vi "Report read csv G.vi"(2 "error in":errorcluster) -> (0 "error out":errorcluster)   [LabVIEW 2015]
uses:
  <vilib>/Utility/file.llb/Read Delimited Spreadsheet (string).vi
  <vilib>/Utility/miscctls.llb/LVRowAndColumnTypeDef.ctl
panel:
  out "Table Control":string[][](table)
  in  "Exit":bool
  in  "Select Date":u16(ring) items=["Select Date", "10_07_20.csv"]
  in  "Select Model No":u16(ring) items=["Select Model", "Global", "Medium"]
  # "Report Data"
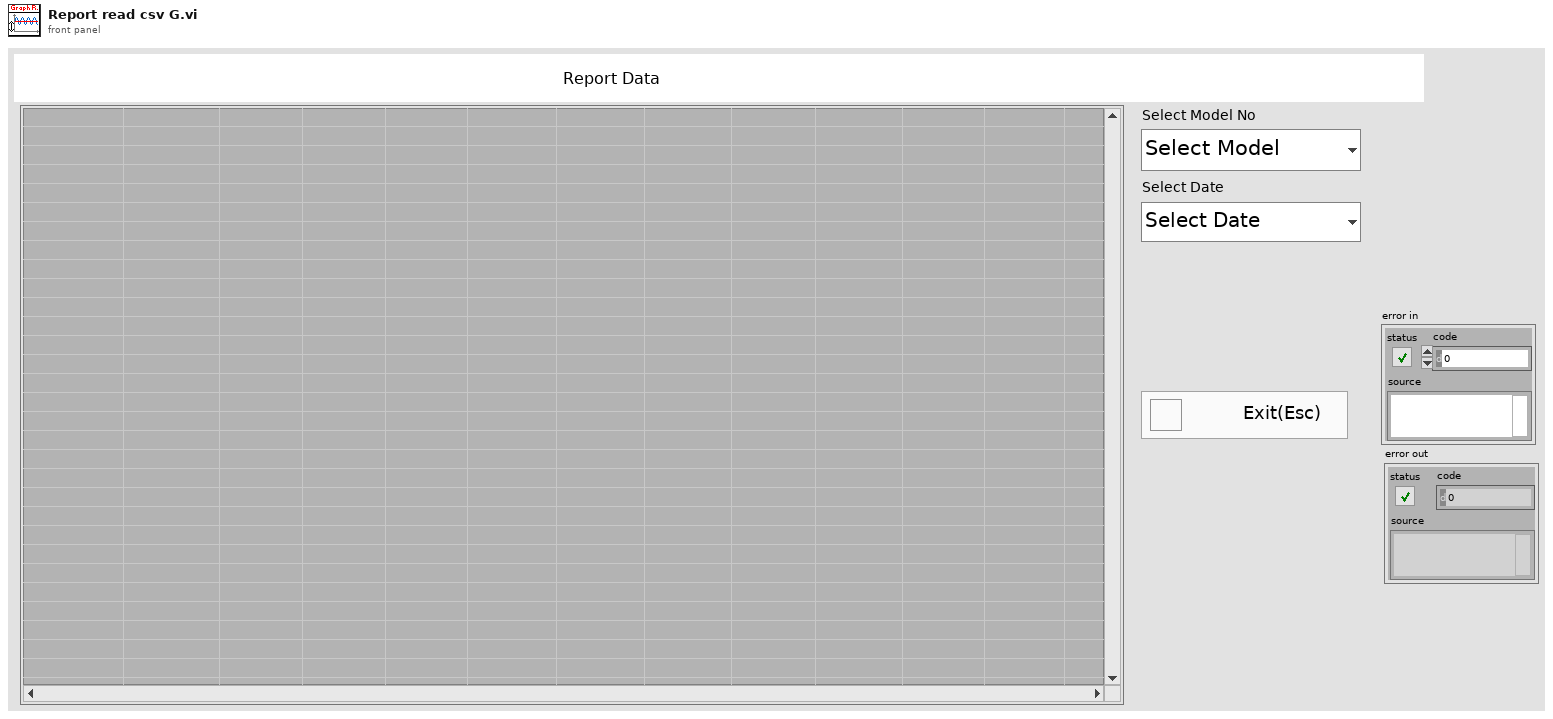
[diagram p1: front panel]
types:
  T1 = typedef "LVRowAndColumnTypeDef.ctl" = cluster{"Row":i32, "Column":i32}
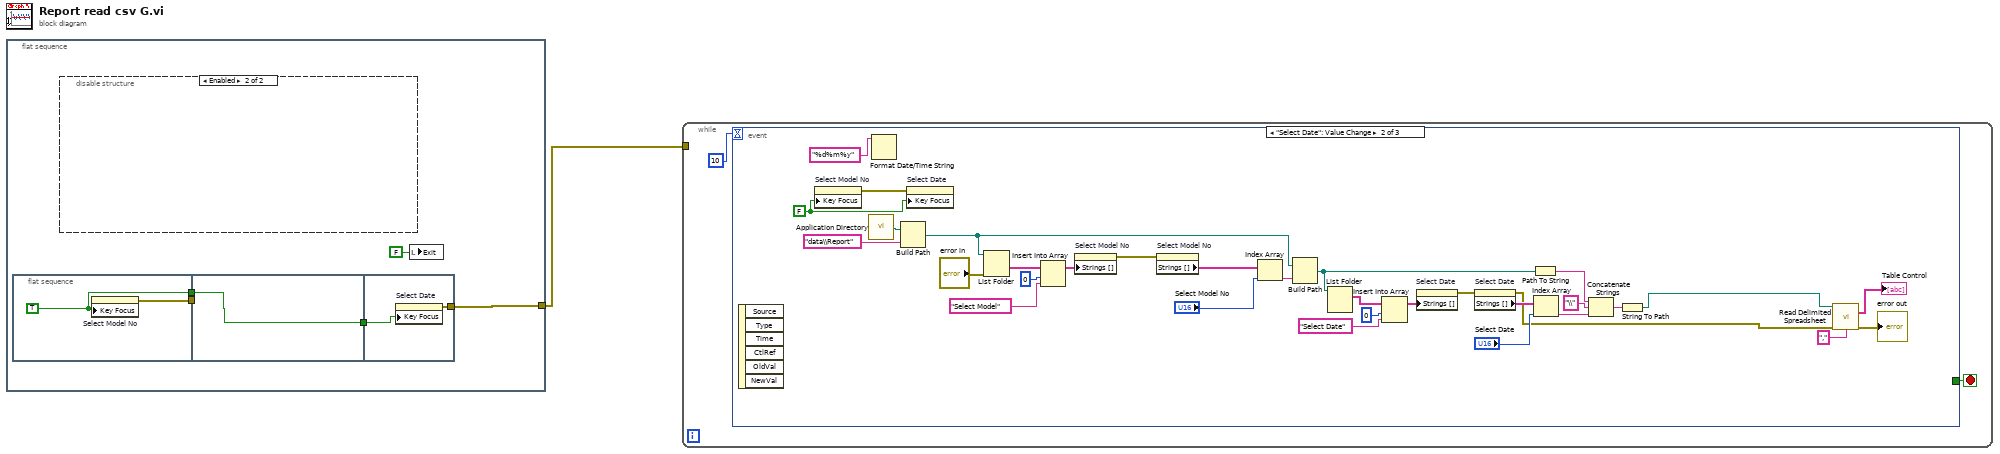
[diagram p0: block diagram]
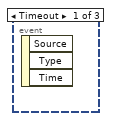
[diagram p2: hidden frame]
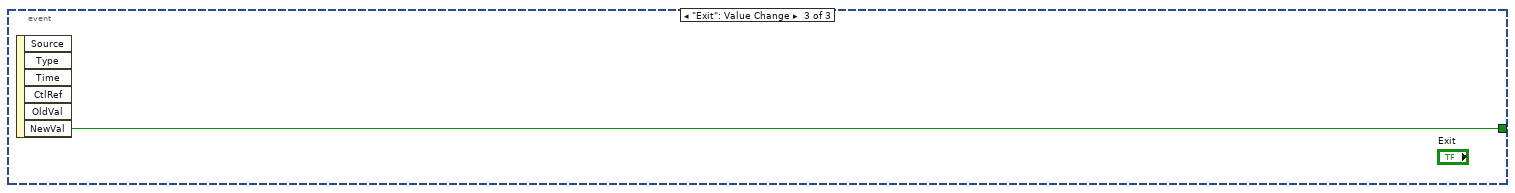
[diagram p3: hidden frame]
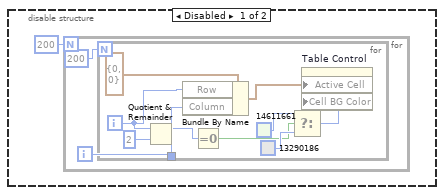
[diagram p4: hidden frame]
diagram:
  n1 = flat-sequence {
    tunnel: [w3] -> w1
    frame #0 {
      n2 = flat-sequence {
        tunnel: [w21] -> w6
        tunnel: [w20] -> w5
        tunnel: w6 -> [_]
        tunnel: w5 -> [w22]
        tunnel: [w22] -> w4
        tunnel: w4 -> [w24]
        tunnel: [w23] -> w3
        frame #0 {
          w20 = TRUE
          n3 = property on="Select Model No" class="Ring (strict)"("Key Focus"=w20) -> (error out=w21:errorcluster)  [unwired: 2 in, 1 out]
        }
        frame #1 {
        }
        frame #2 {
          n4 = property on="Select Date" class="Ring (strict)"("Key Focus"=w24) -> (error out=w23:errorcluster)  [unwired: 2 in, 1 out]
        }
      }
      n5 = disable-structure shown="Enabled" {
        frame Disabled {
          n6 = for {
            N: 200 -> [_]
            i -> [w9]
            n7 = for {
              N: 200 -> [_]
              tunnel: w9 -> [w17]
              i -> [w14]
              n8 = Quotient & Remainder(x=w14, y=2) -> (x-y*floor(x/y)=w12:i32)  [unwired: 1 out]
              n9 = Bundle By Name(cluster=T1 {"Row"=0, "Column"=0} ("Active Cell:Active Cell"), "Row"=w14, "Column"=w17) -> (w18:T1)
              n10 = Equal To 0?(x=w12) -> (x = 0?=w11:bool)
              n11 = Select(t=u32 14611661, s=w11, f=u32 13290186) -> (s? t:f=w10:u32)
              n12 = property on="Table Control" class="Tbl (strict)"("Active Cell"=w18, "Cell BG Color"=w10) -> ()  [unwired: 2 in, 2 out]
            }
          }
        }
        frame Enabled {
        }
      }
      n13 = local write "Exit"(FALSE ("Exit")) -> ()
    }
  }
  n14 = while {
    tunnel: w1 -> [_]
    stop <- w25 stop-if-true
    n15 = event shown="[1] \"Select Date\": Value Change" {
      selector: _ -> [_ _ _]
      dyn-events: _ -> [_ _ _]
      timeout: 10 -> [_ _ _]
      tunnel: [_ _ w59] -> w25
      event Timeout {
        n16 = event-data() -> ()  [unwired: 1 in, 3 out]
      }
      event "Select Date": Value Change {
        w41 = FALSE
        n17 = event-data() -> ()  [unwired: 1 in, 6 out]
        n18 = property on="Select Model No" class="Ring (strict)"("Key Focus"=w41) -> (error out=w35:errorcluster)  [unwired: 2 in, 1 out]
        n19 = call <vilib>:"Application Directory.vi"() -> ("Application Directory"=w39:path)
        n20 = Format Date/Time String(time format string (%c)="%d%m%y") -> ()  [unwired: 2 in, 1 out]
        n21 = Build Path(base path=w39, name or relative path="data\\Report") -> (appended path=w37:path)
        n22 = property on="Select Date" class="Ring (strict)"(error in=w35, "Key Focus"=w41) -> ()  [unwired: 1 in, 2 out]
        n23 = List Folder(path=w37, error in="error in") -> (folder names=w57:string[])  [unwired: 2 in, 3 out]
        n24 = Insert Into Array(array=w57, index=0, new element="Select Model" ("string")) -> (w55:string[])
        n25 = property on="Select Model No" class="Ring (strict)"("Strings []"=w55) -> (error out=w54:errorcluster)  [unwired: 2 in, 1 out]
        n26 = property on="Select Model No" class="Ring (strict)"(error in=w54) -> ("Strings []"=w53:string[])  [unwired: 1 in, 2 out]
        n27 = Index Array(array=w53, index="Select Model No") -> (element=w36:string)
        n28 = Build Path(base path=w37, name or relative path=w36) -> (appended path=w33:path)
        n29 = List Folder(path=w33) -> (filenames=w31:string[])  [unwired: 3 in, 3 out]
        n30 = Insert Into Array(array=w31, index=0, new element="Select Date" ("string")) -> (w49:string[])
        n31 = property on="Select Date" class="Ring (strict)"("Strings []"=w49) -> (error out=w48:errorcluster)  [unwired: 2 in, 1 out]
        n32 = property on="Select Date" class="Ring (strict)"(error in=w48) -> (error out=w29:errorcluster, "Strings []"=w46:string[])  [unwired: 1 in, 1 out]
        n33 = Path To String(path=w33) -> (string=w32:string)
        n34 = Index Array(array=w46, index="Select Date") -> (element=w44:string)
        n35 = Concatenate Strings(w32, "\\" ("string"), w44) -> (w45:string)
        n36 = String To Path(string=w45) -> (path=w30:path)
        n37 = call-poly <vilib>:"Read Delimited Spreadsheet.vi"("file path (dialog if empty)"=w30, "error in (no error)"=w29, "delimiter (\\t)"="," ("delimiter (\\t)")) -> ("all rows"=→"Table Control":string[][], "error out"=→"error out":errorcluster)  [unwired: 7 in, 4 out]
      }
      event "Exit": Value Change {
        n38 = event-data() -> ("NewVal"=w59:bool)  [unwired: 1 in, 5 out]
      }
    }
  }
